vi "Shift_002.vi"() -> ()   [LabVIEW 2019]
panel:
  out "a":dbl[unit][](graph)
  out "v":dbl[unit][](graph)
  out "x":dbl[unit][](graph)
  out "x(tk)":dbl[unit][](array[numeric])
  out "v(tk)":dbl[unit][](array[numeric])
  out "a(k)":dbl[unit][](array[numeric])
  in  "M":dbl[unit]
  in  "k":dbl[unit]
  in  "v0":dbl[unit]
  in  "x0":dbl[unit]
  in  "Dt":dbl[unit]=1e-05
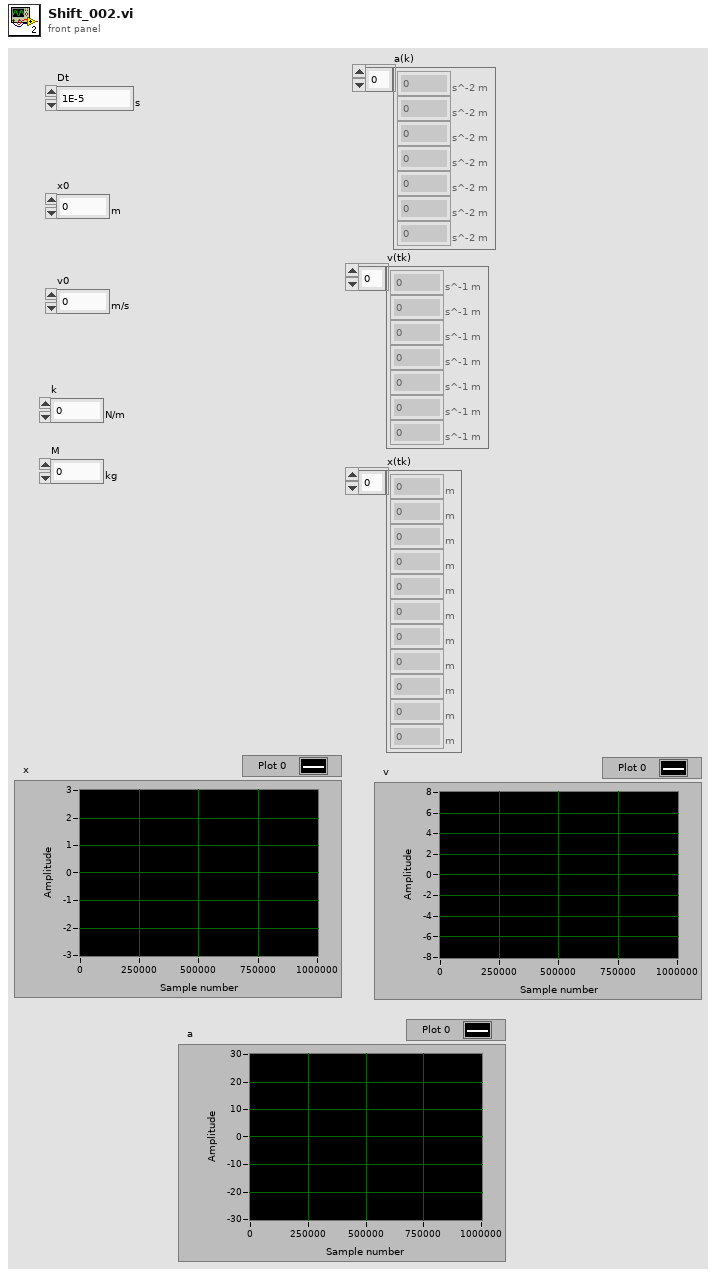
[diagram p1: front panel]
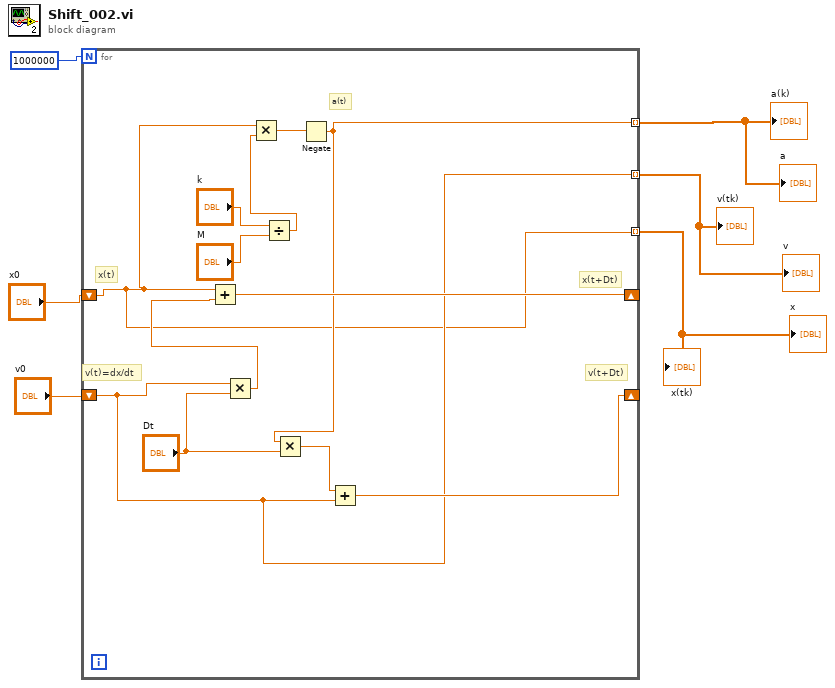
[diagram p0: block diagram]
diagram:
  n1 = for {
    N: 1000000 -> [_]
    shift-right: [w17] -> _
    shift-left: "x0" -> [w7]
    shift-right: [w10] -> _
    shift-left: "v0" -> [w8]
    tunnel: [w9] -> w3 mode=indexing
    tunnel: [w8] -> w2 mode=indexing
    tunnel: [w7] -> w1 mode=indexing
    # "a(t)"
    # "v(t+Dt)"
    # "x(t+Dt)"
    # "v(t)=dx/dt"
    # "x(t)"
    n2 = Multiply(x=w8, y="Dt") -> (x*y=w18:dbl[unit])
    n3 = Add(x=w7, y=w18) -> (x+y=w17:dbl[unit])
    n4 = Divide(x="k", y="M") -> (x/y=w14:dbl[unit])
    n5 = Multiply(x=w7, y=w14) -> (x*y=w13:dbl[unit])
    n6 = Negate(x=w13) -> (-x=w9:dbl[unit])
    n7 = Multiply(x=w9, y="Dt") -> (x*y=w11:dbl[unit])
    n8 = Add(x=w11, y=w8) -> (x+y=w10:dbl[unit])
  }
  "a(k)" <- w3
  "v(tk)" <- w2
  "x(tk)" <- w1
  "v" <- w2
  "a" <- w3
  "x" <- w1
